vi "Simulations Config.vi"(8 "error in (no error)":errorcluster, 11 "Config in":refnum<class "Config.lvclass">) -> (0 "error out":errorcluster, 1 "Found?":bool, 2 "Simulated Classes":T1, 3 "Config out":refnum<class "Config.lvclass">)   [LabVIEW 2019, in "Config.lvlib" / "Config.lvclass"]
doc: "This method reads the simulation constants for the file. The default values are all not simulated."
uses:
  Config.lvclass
  Controls/Simulated Classes.ctl
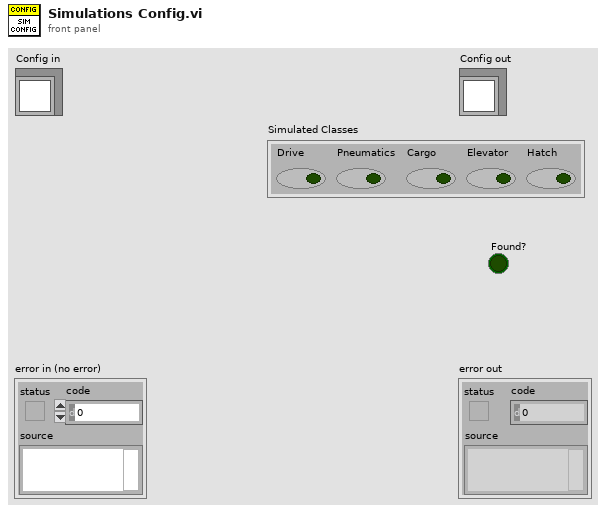
[diagram p1: front panel]
types:
  T1 = typedef "Config.lvlib/Config.lvclass/Simulated Classes.ctl" = cluster{"Drive":bool, "Pneumatics":bool, "Cargo":bool, "Elevator":bool, "Hatch":bool}
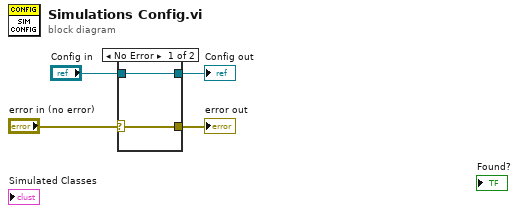
[diagram p0: block diagram]
diagram:
  n1 = case shown="No Error" "error in (no error)" {
    selector: "error in (no error)" -> [w5 w8]
    tunnel: [w5 w8] -> w3
    tunnel: [w6 w7] -> w1
    tunnel: "Config in" -> [w6 w7]
    frame No Error {
    }
    frame Error {
    }
  }
  "error out" <- w3
  "Config out" <- w1
